vi "AddModel.vi"(8 "error in":errorcluster caption="错误输入", 11 "Setup":T1) -> (0 "error out":errorcluster caption="错误输出")   [LabVIEW 2013]
uses:
  SetupCtl.ctl
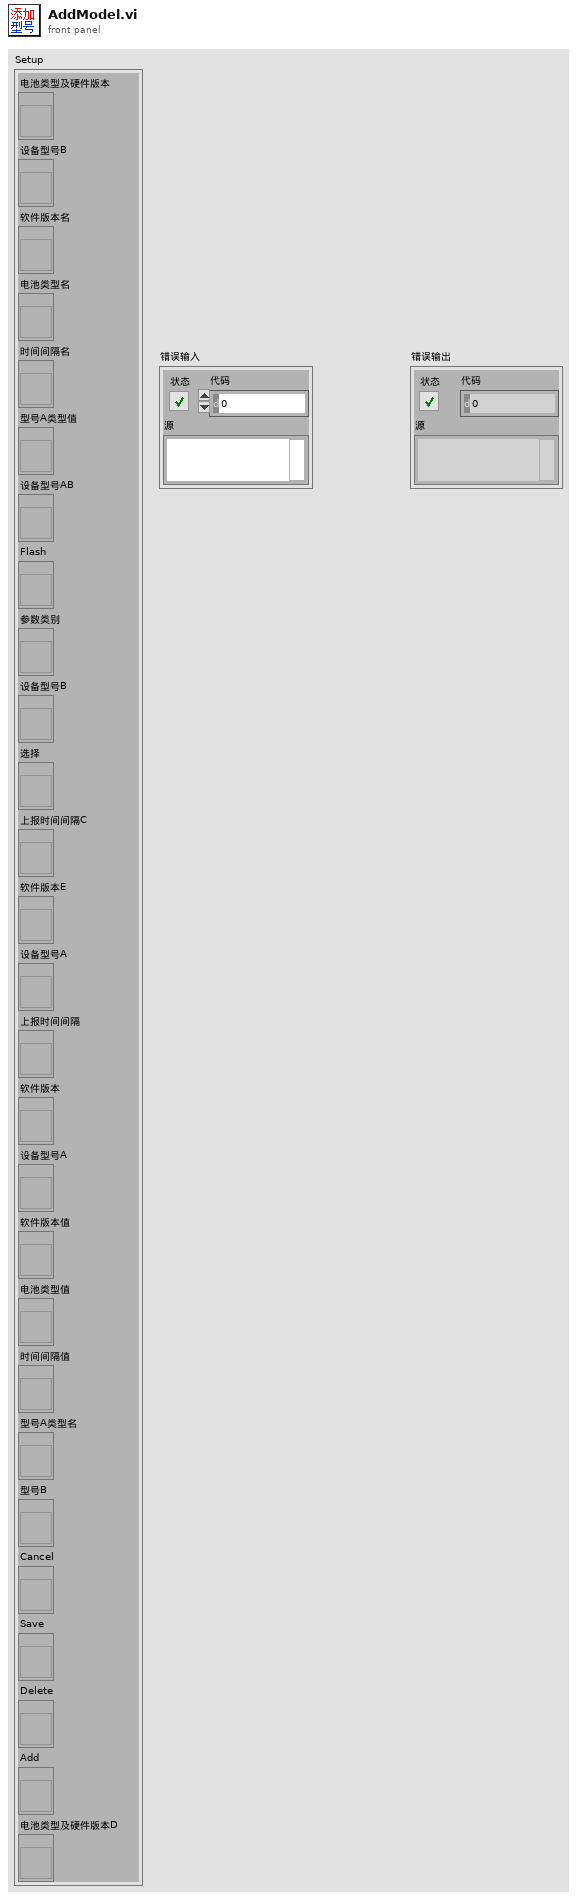
[diagram p1: front panel]
types:
  T1 = typedef "SetupCtl.ctl" = cluster{"电池类型及硬件版本":refnum<vi>, "设备型号B":refnum<vi>, "软件版本名":refnum<vi>, "电池类型名":refnum<vi>, "时间间隔名":refnum<vi>, "型号A类型值":refnum<vi>, "设备型号AB":refnum<vi>, "Flash":refnum<vi>, "参数类别":refnum<vi>, "设备型号B":refnum<vi>, "选择":refnum<vi>, "上报时间间隔C":refnum<vi>, "软件版本E":refnum<vi>, "设备型号A":refnum<vi>, "上报时间间隔":refnum<vi>, "软件版本":refnum<vi>, "设备型号A":refnum<vi>, "软件版本值":refnum<vi>, "电池类型值":refnum<vi>, "时间间隔值":refnum<vi>, "型号A类型名":refnum<vi>, "型号B":refnum<vi>, "Cancel":refnum<vi>, "Save":refnum<vi>, "Delete":refnum<vi>, "Add":refnum<vi>, "电池类型及硬件版本D":refnum<vi>}
  T2 = enum16{"型号A类型名", "型号A类型值", "型号B", "时间间隔名", "时间间隔值", "电池类型名", "电池类型值", "软件版本名", "软件版本值"}
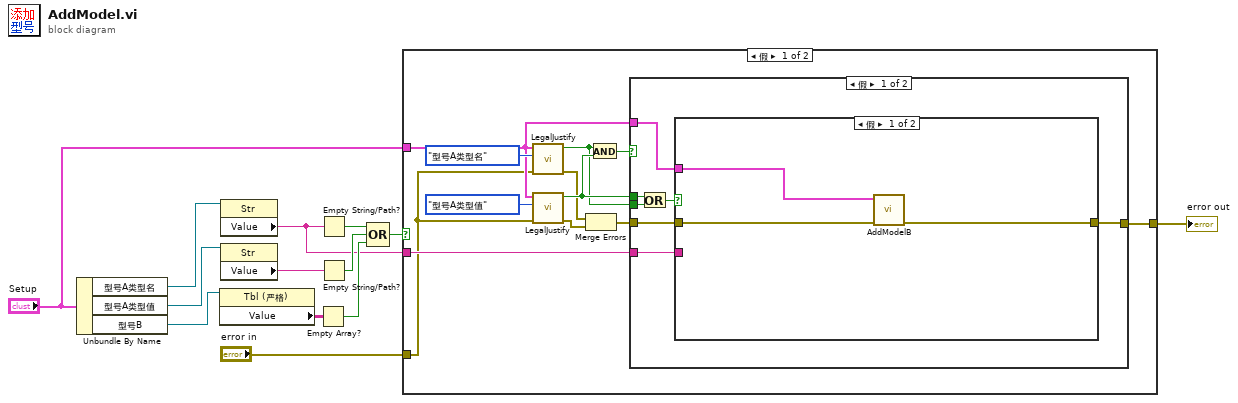
[diagram p0: block diagram]
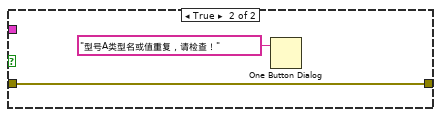
[diagram p2: hidden frame]
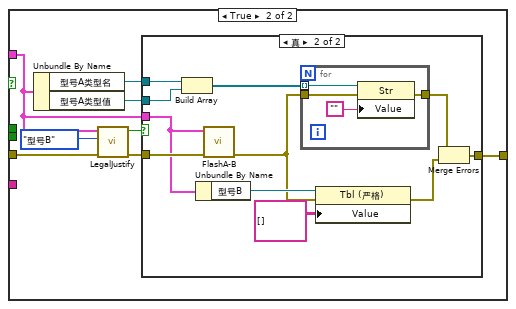
[diagram p3: hidden frame]
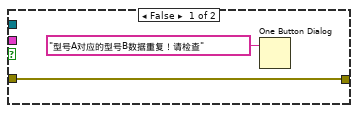
[diagram p4: hidden frame]
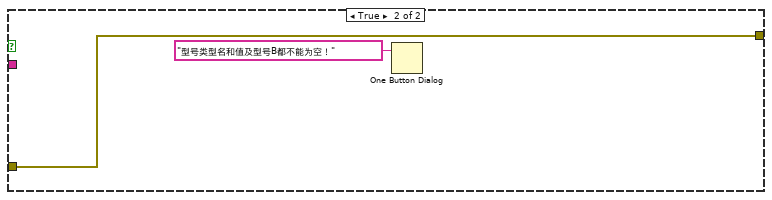
[diagram p5: hidden frame]
diagram:
  n1 = Unbundle By Name("Setup") -> ("型号A类型名"=w13:refnum<vi>, "型号A类型值"=w12:refnum<vi>, "型号B"=w11:refnum<vi>)
  n2 = property class="Tbl (严格)"(reference=w11) -> ("Value"=w9:string[][])  [unwired: 1 in, 2 out]
  n3 = property class="Str"(reference=w13) -> ("Value"=w3:string)  [unwired: 1 in, 2 out]
  n4 = property class="Str"(reference=w12) -> ("Value"=w10:string)  [unwired: 1 in, 2 out]
  n5 = Empty Array?(array=w9) -> (empty?=w6:bool)
  n6 = Empty String/Path?(string/path=w3) -> (empty?=w8:bool)
  n7 = Empty String/Path?(string/path=w10) -> (empty?=w7:bool)
  n8 = Compound Arithmetic op=OR(w8, w7, w6) -> (w5:bool)
  n9 = case shown="假" w5 {
    tunnel: "Setup" -> [w22 _]
    tunnel: w3 -> [w19 _]
    tunnel: "error in" -> [w18 w63]
    tunnel: [w14 w63] -> w1
    frame False {
      n10 = call "LegalJustify.vi"("error in"=w18, "JustifyName"=T2."型号A类型名", "Setup"=w22) -> ("error out"=w17:errorcluster, "OK？"=w20:bool)  [unwired: 7 in]
      n11 = call "LegalJustify.vi"("error in"=w18, "JustifyName"=T2."型号A类型值", "Setup"=w22) -> ("error out"=w16:errorcluster, "OK？"=w21:bool)  [unwired: 7 in]
      n12 = Merge Errors(w17, w16) -> (w15:errorcluster)
      n13 = And(x=w20, y=w21) -> (x .and. y?=w23:bool)
      n14 = case shown="假" w23 {
        tunnel: w22 -> [w28 w41]
        tunnel: w21 -> [w32 _]
        tunnel: w20 -> [w31 _]
        tunnel: w19 -> [w29 _]
        tunnel: w15 -> [w27 w42]
        tunnel: [w26 w38] -> w14
        frame False {
          n15 = Or(x=w32, y=w31) -> (x .or. y?=w30:bool)
          n16 = case shown="假" w30 {
            tunnel: w29 -> [_ _]
            tunnel: w28 -> [w35 _]
            tunnel: w27 -> [w34 w36]
            tunnel: [w33 w36] -> w26
            frame False {
              n17 = call "AddModelB.vi"("error in"=w34, "Setup"=w35) -> ("error out"=w33:errorcluster)  [unwired: 9 in]
            }
            frame True {
              n18 = One Button Dialog(message="型号A类型名或值重复，请检查！" ("消息")) -> ()  [unwired: 1 in, 1 out]
            }
          }
        }
        frame True {
          n19 = Unbundle By Name(w41) -> ("型号A类型名"=w40:refnum<vi>, "型号A类型值"=w39:refnum<vi>)
          n20 = call "LegalJustify.vi"("error in"=w42, "JustifyName"=T2."型号B", "Setup"=w41) -> ("error out"=w43:errorcluster, "OK？"=w44:bool)  [unwired: 7 in]
          n21 = case shown="真" w44 {
            tunnel: w41 -> [_ w54]
            tunnel: w43 -> [w46 w58]
            tunnel: w40 -> [_ w57]
            tunnel: w39 -> [_ w56]
            tunnel: [w46 w48] -> w38
            frame False {
              n22 = One Button Dialog(message="型号A对应的型号B数据重复！请检查" ("消息")) -> ()  [unwired: 1 in, 1 out]
            }
            frame True {
              n23 = Build Array(w57, w56) -> (w55:refnum<vi>[])
              n24 = Unbundle By Name(w54) -> ("型号B"=w53:refnum<vi>)
              n25 = call "FlashA-B.vi"("error in"=w58, "Setup"=w54) -> ("error out"=w52:errorcluster)  [unwired: 9 in]
              n26 = for {
                tunnel: w55 -> [w62] mode=indexing
                tunnel: w52 -> [w60]
                tunnel: [w59] -> w50
                n27 = property class="Str"(reference=w62, error in=w60, "Value"="") -> (error out=w59:errorcluster)  [unwired: 1 out]
              }
              n28 = property class="Tbl (严格)"(reference=w53, error in=w52, "Value"=string[][] [] ("值")) -> (error out=w49:errorcluster)  [unwired: 1 out]
              n29 = Merge Errors(w50, w49) -> (w48:errorcluster)
            }
          }
        }
      }
    }
    frame True {
      n30 = One Button Dialog(message="型号类型名和值及型号B都不能为空！" ("消息")) -> ()  [unwired: 1 in, 1 out]
    }
  }
  "error out" <- w1
